vi "DAQmx.GetPublicEvents.vi"(8 "error in (no error)":errorcluster, 11 "DAQmx":refnum<class "DAQmx.lvclass">) -> (0 "error out":errorcluster, 2 "DAQmx Public Events":T1, 3 "DAQmx out":refnum<class "DAQmx.lvclass">)   [LabVIEW 2019, in "DAQmx.lvclass"]
doc: "---------------------------------------------------------------\nJKI State Machine Objects™\nhttp://jki.net/state-machine-objects/\nCopyright (C) 2005-2015, JKI <info@jki.net>\nALL RIGHTS RESERVEDJKI State Machine Objects (SMO) 1.0.0.4\nJKI - JKI\nCopyright (c) 2015, JKI"
uses:
  DAQmx.lvclass
  typedefs/PublicEvents--Cluster.ctl
  typedefs/DAQmx.Status--enum.ctl
  typedefs/DeviceInfo--Cluster.ctl
  typedefs/DAQ.Config.Timing.Sampling--Cluster.ctl
  typedefs/DAQ.Config.AO--Cluster--Array.ctl
  typedefs/DAQ.Config.AO--Cluster.ctl
  typedefs/DAQ.Config.AO.Range--enum.ctl
  typedefs/DAQ.Config.Device Type--enum.ctl
  typedefs/DAQ.Config.AI--Cluster--Array.ctl
  typedefs/DAQ.Config.AI--Cluster.ctl
  typedefs/DAQ.Config.AI.Coupling--enum.ctl
  typedefs/DAQ.Config.AI.Range--enum.ctl
  typedefs/PrivateEvent--Waveforms--cluster.ctl
  DAQmx.lvclass/DAQmx.ctl
panel:
  # "For instructions on how to use the JKI State Machine Objects, examples and video tutorials, visit:\nhttp://jki.net/state-machine-objects/\n\nJKI State Machine Objects™\nhttp://jki.net/state-machine-objects/\nCopyright (C) 2005-2015, JKI <info@jki.net>\nALL RIGHTS RESERVED"
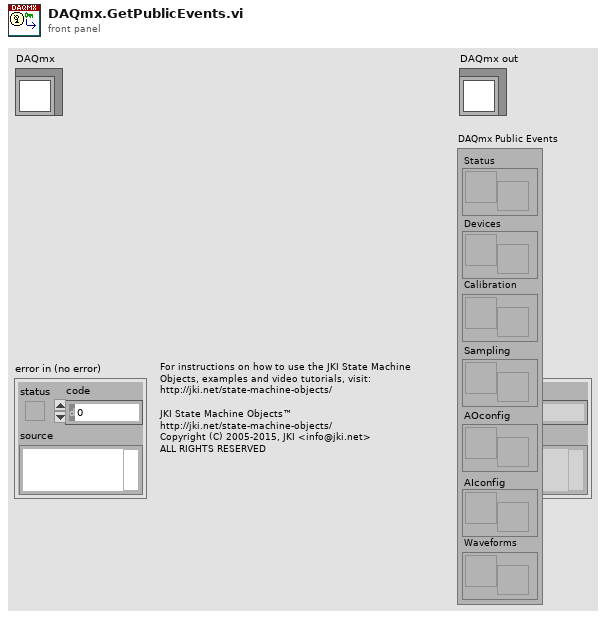
[diagram p1: front panel]
types:
  T1 = typedef "DAQmx.lvclass/PublicEvents--Cluster.ctl" = cluster{"Status":refnum<user-event>, "Devices":refnum<user-event>, "Calibration":refnum<user-event>, "Sampling":refnum<user-event>, "AOconfig":refnum<user-event>, "AIconfig":refnum<user-event>, "Waveforms":refnum<user-event>}
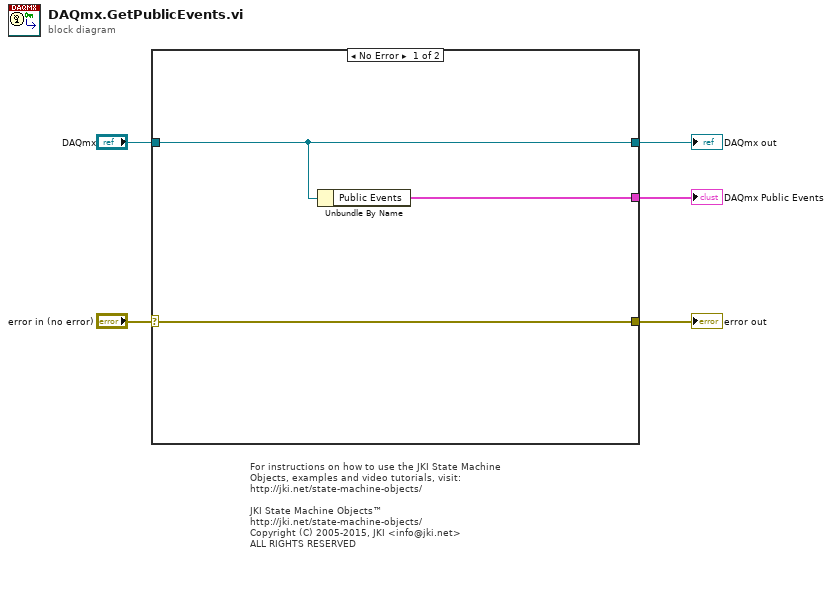
[diagram p0: block diagram]
diagram:
  # "For instructions on how to use the JKI State Machine Objects, examples and video tutorials, visit:\nhttp://jki.net/state-machine-objects/\n\nJKI State Machine Objects™\nhttp://jki.net/state-machine-objects/\nCopyright (C) 2005-2015, JKI <info@jki.net>\nALL RIGHTS RESERVED"
  n1 = case shown="No Error" "error in (no error)" {
    selector: "error in (no error)" -> [w7 w9]
    tunnel: "DAQmx" -> [w6 w10]
    tunnel: [w7 w9] -> w4
    tunnel: [w6 w10] -> w3
    tunnel: [w8 _] -> w1
    frame No Error {
      n2 = Unbundle By Name(w6) -> ("Public Events"=w8:T1)
    }
    frame Error {
    }
  }
  "error out" <- w4
  "DAQmx out" <- w3
  "DAQmx Public Events" <- w1
